vi "Write Author Table.vi"(8 "Error In":errorcluster, 11 "Database Full Information In":T1 {"Database Write Information"."Layer Information Array"."Deposition Method" items=["Blade Coating", "Spin Coating", "Thermal Evaporation", "E-Beam Evaporation", "Sputtering", "Drop Casting", "Dip Coating", "Pulsed Laser Deposition", "Chemival Vapour Deposition", "Atomic Layer Deposition", "Spray Coating", "Screen Printing", "Electroplating", "Molecular Beam Epitaxy", "Custom Deposition"]; "Database Write Information"."Layer Information Array"."Layer Type" items=["Front Electrode", "Electron Transport Layer", "Active Layer", "Hole Transport Layer", "Back Electrode", "Custom Layer"]}) -> (0 "Error Out":errorcluster, 3 "Database Full Information Out":T1 {"Database Write Information"."Layer Information Array"."Deposition Method" items=["Blade Coating", "Spin Coating", "Thermal Evaporation", "E-Beam Evaporation", "Sputtering", "Drop Casting", "Dip Coating", "Pulsed Laser Deposition", "Chemival Vapour Deposition", "Atomic Layer Deposition", "Spray Coating", "Screen Printing", "Electroplating", "Molecular Beam Epitaxy", "Custom Deposition"]; "Database Write Information"."Layer Information Array"."Layer Type" items=["Front Electrode", "Electron Transport Layer", "Active Layer", "Hole Transport Layer", "Back Electrode", "Custom Layer"]})   [LabVIEW 2020]
uses:
  Data Clusters/Database Information.ctl
  Data Clusters/Layer Information Cluster.ctl
  <vilib>/addons/database/Connection.llb/Conn ObjectReference.ctl
  <vilib>/addons/database/NI_Database_API.lvlib
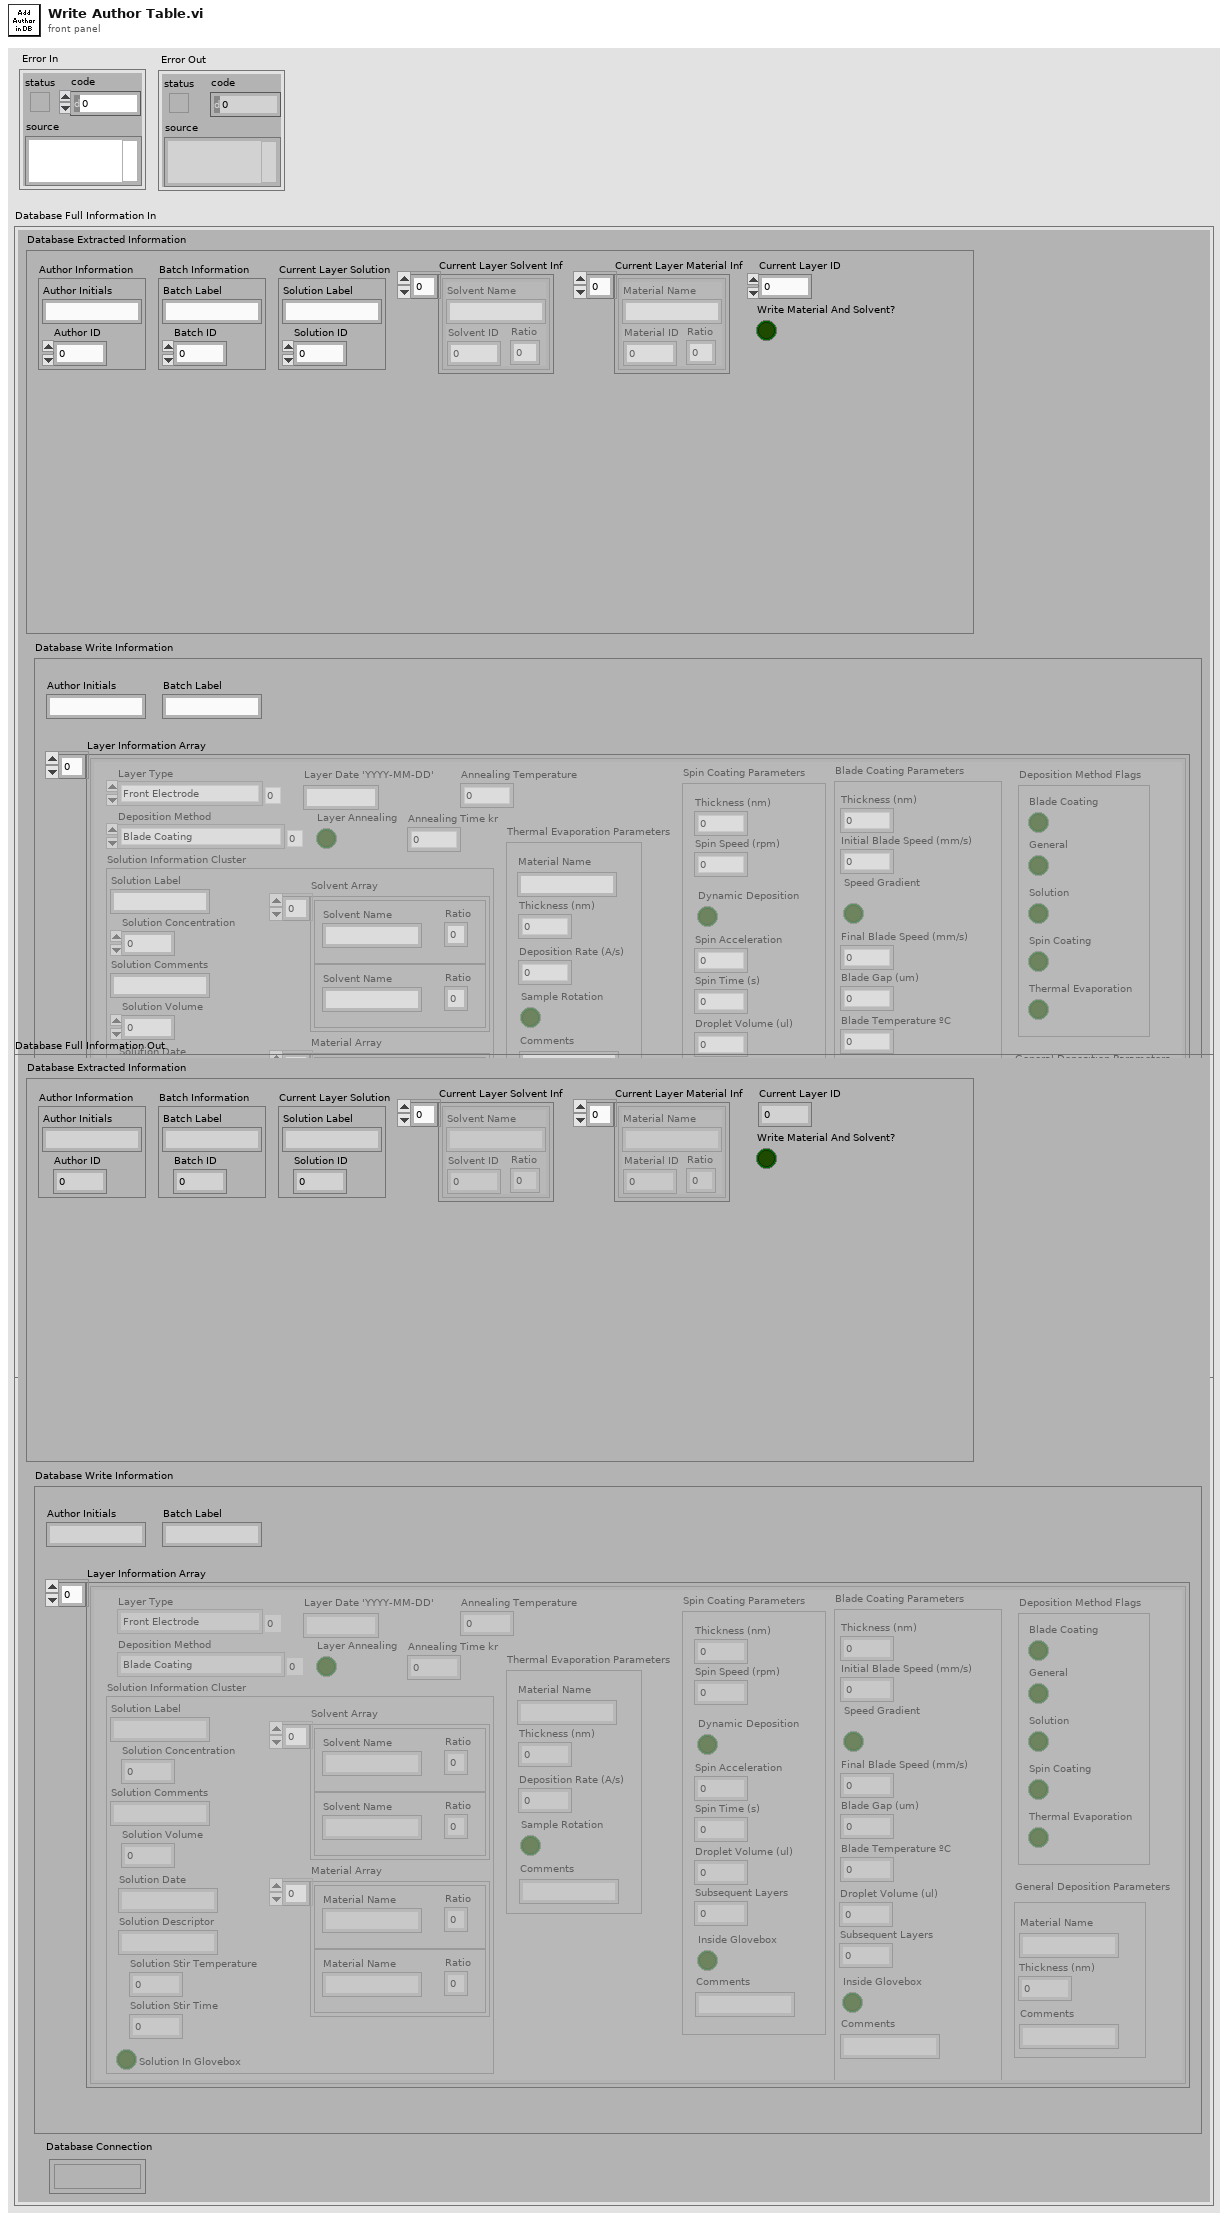
[diagram p1: front panel]
types:
  T1 = typedef "Database Information.ctl" = cluster{"Database Extracted Information":cluster{"Author Information":cluster{"Author Initials":string, "Author ID":i32}, "Batch Information":cluster{"Batch Label":string, "Batch ID":i32}, "Current Layer Solution":cluster{"Solution Label":string, "Solution ID":i32}, "Current Layer ID":i32, "Current Layer Solvent Inf":cluster{"Solvent Name":string, "Solvent ID":i32, "Ratio":dbl}[], "Current Layer Material Inf":cluster{"Material Name":string, "Material ID":i32, "Ratio":dbl}[], "Write Material And Solvent?":bool}, "Database Write Information":cluster{"Author Initials":string, "Batch Label":string, "Layer Information Array":T2[]}, "Database Connection":T3}
  T2 = typedef "Layer Information Cluster.ctl" = cluster{"Solution Information Cluster":cluster{"Solution Label":string, "Solution Concentration":dbl, "Solution Comments ":string, "Solution Volume ":dbl, "Solution Date ":string, "Solution Descriptor ":string, "Solution Stir Temperature ":dbl, "Solution Stir Time ":dbl, "Solution In Glovebox":bool, "Solvent Array":cluster{"Solvent Name":string, "Ratio":dbl}[], "Material Array":cluster{"Material Name":string, "Ratio":dbl}[]}, "Layer Type":u16, "Deposition Method":u16, "Layer Annealing":bool, "General Deposition Parameters":cluster{"Thickness (nm)":dbl, "Comments":string, "Material Name":string}, "Blade Coating Parameters":cluster{"Thickness (nm)":dbl, "Initial Blade Speed (mm/s)":dbl, "Speed Gradient":bool, "Final Blade Speed (mm/s)":dbl, "Blade Gap (um)":dbl, "Droplet Volume (ul)":dbl, "Subsequent Layers":dbl, "Inside Glovebox":bool, "Comments":string, "Blade Temperature ºC":dbl}, "Spin Coating Parameters":cluster{"Thickness (nm)":dbl, "Spin Speed (rpm)":dbl, "Dynamic Deposition":bool, "Spin Acceleration":dbl, "Spin Time (s)":dbl, "Droplet Volume (ul)":dbl, "Subsequent Layers":dbl, "Inside Glovebox":bool, "Comments":string}, "Thermal Evaporation Parameters":cluster{"Deposition Rate (A/s)":dbl, "Thickness (nm)":dbl, "Comments":string, "Material Name":string, "Sample Rotation":bool}, "Layer Date 'YYYY-MM-DD'":string, "Annealing Time kr":dbl, "Annealing Temperature":dbl, "Deposition Method Flags":cluster{"Blade Coating":bool, "General ":bool, "Solution":bool, "Spin Coating":bool, "Thermal Evaporation":bool}}
  T3 = typedef "NI_Database_API.lvlib/Conn ObjectReference.ctl" = refnum<k1>
  T4 = cluster{"Author Initials":string, "Author ID":i32}
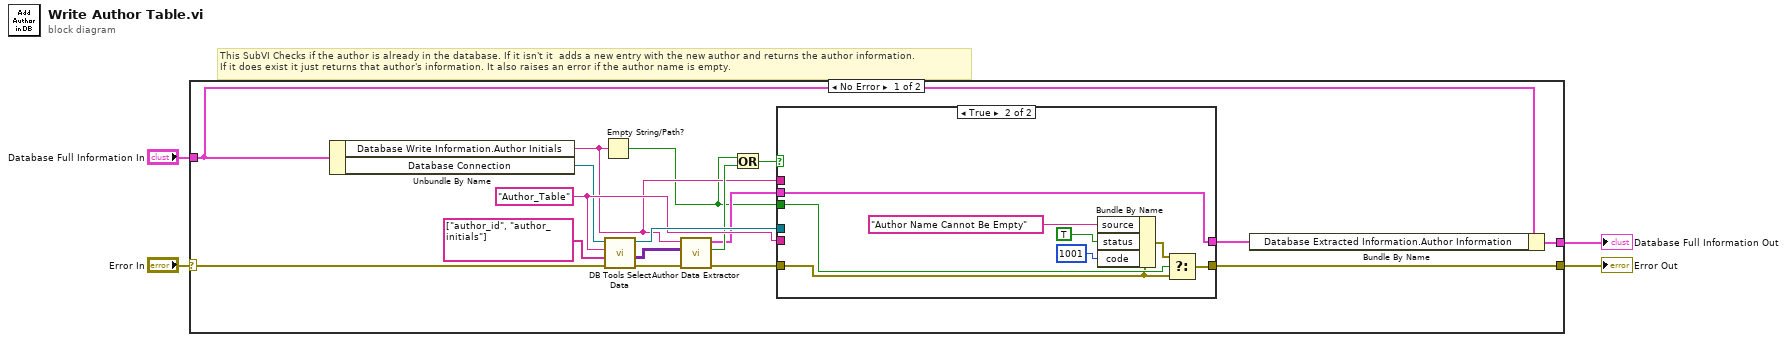
[diagram p0: block diagram]
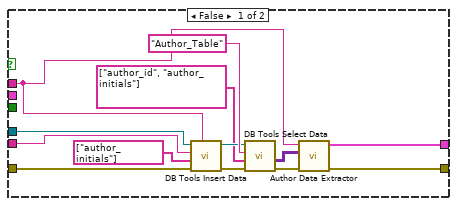
[diagram p2: hidden frame]
diagram:
  # "This SubVI Checks if the author is already in the database. If it isn't it  adds a new entry with the new author and returns the author information.\nIf it does exist it just returns that author's information. It also raises an error if the author name is empty."
  n1 = case shown="No Error" "Error In" {
    selector: "Error In" -> [w18 w44]
    tunnel: [w17 w44] -> w3
    tunnel: "Database Full Information In" -> [w9 w43]
    tunnel: [w7 w43] -> w1
    frame No Error {
      w19 = "Author_Table" ("table")
      n2 = Unbundle By Name(w9) -> ("Database Write Information.Author Initials"=w10:string, "Database Connection"=w6:T3)
      n3 = Empty String/Path?(string/path=w10) -> (empty?=w5:bool)
      n4 = call <vilib>:"DB Tools Select Data.vi"("error in (no error)"=w18, "columns"=string[] ["author_id", "author_initials"], "table"=w19, "connection reference"=w6) -> ("error out"=w14:errorcluster, "data"=w15:variant[][], "connection reference out"=w21:T3)  [unwired: 2 in]
      n5 = call "Author Data Extractor.vi"("Error In"=w14, "Author Data"=w15, "Author Initials"=w10) -> ("Error Out"=w12:errorcluster, "Exists?"=w13:bool, "Author Information"=w11:T4)  [unwired: 6 in]
      n6 = Or(x=w5, y=w13) -> (x .or. y?=w16:bool)
      n7 = case shown="True" w16 {
        tunnel: w10 -> [w24 _]
        tunnel: w12 -> [w34 w35]
        tunnel: w21 -> [w33 _]
        tunnel: w19 -> [w32 _]
        tunnel: [w22 w36] -> w17
        tunnel: w11 -> [_ w42]
        tunnel: [w23 w42] -> w8
        tunnel: w5 -> [_ w38]
        frame False {
          n8 = call <vilib>:"DB Tools Insert Data.vi"("data"=w24, "error in (no error)"=w34, "columns"=string[] ["author_initials"], "table"=w32, "connection reference"=w33) -> ("error out"=w26:errorcluster, "connection reference out"=w29:T3)  [unwired: 5 in]
          n9 = call <vilib>:"DB Tools Select Data.vi"("error in (no error)"=w26, "columns"=string[] ["author_id", "author_initials"], "table"="Author_Table", "connection reference"=w29) -> ("error out"=w25:errorcluster, "data"=w27:variant[][])  [unwired: 2 in, 1 out]
          n10 = call "Author Data Extractor.vi"("Error In"=w25, "Author Data"=w27, "Author Initials"=w24) -> ("Error Out"=w22:errorcluster, "Author Information"=w23:T4)  [unwired: 6 in, 1 out]
        }
        frame True {
          n11 = Bundle By Name(cluster=w35, "source"="Author Name Cannot Be Empty", "status"=TRUE, "code"=1001) -> (w37:errorcluster)
          n12 = Select(t=w37, s=w38, f=w35) -> (s? t:f=w36:errorcluster)
        }
      }
      n13 = Bundle By Name(cluster=w9, "Database Extracted Information.Author Information"=w8) -> (w7:T1)
    }
    frame Error {
    }
  }
  "Error Out" <- w3
  "Database Full Information Out" <- w1
